vi "TrackExtractor2.vi"() -> ()   [LabVIEW 2012]
panel:
  out "error out":errorcluster
  in  "Tracking file":path=path "C:/Users/Ludovico/Lavoro/Experiments/Autofocus/vermi/track3.txt"
  in  "Positions file":path=path "C:/Users/Ludovico/Lavoro/Experiments/Autofocus/vermi/CONFSTAGELOG/2016_12_16_10_06.txt"
  in  "error in (no error)":errorcluster
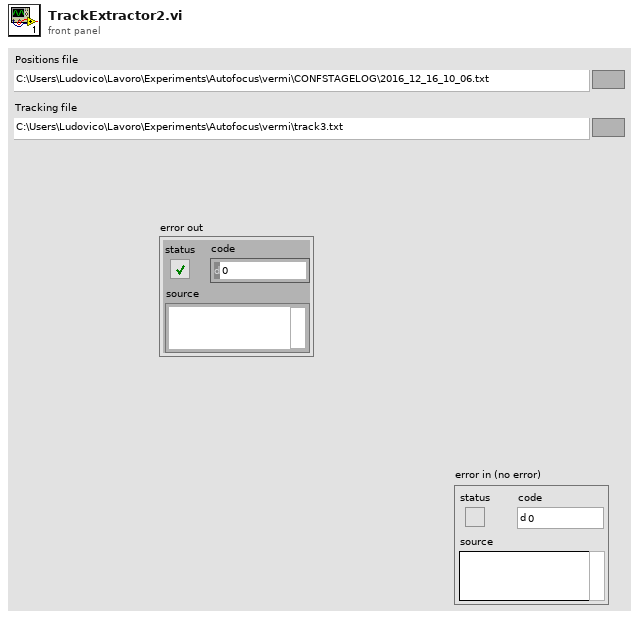
[diagram p1: front panel]
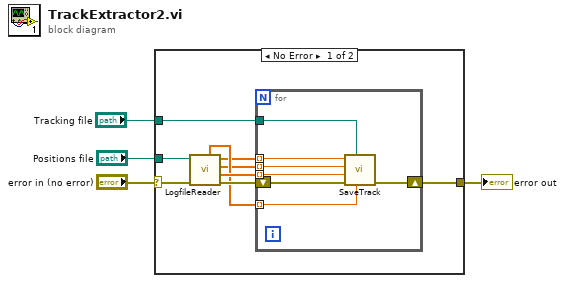
[diagram p0: block diagram]
diagram:
  n1 = case shown="No Error" "error in (no error)" {
    selector: "error in (no error)" -> [w13 w21]
    tunnel: "Positions file" -> [w12 _]
    tunnel: "Tracking file" -> [w6 _]
    tunnel: [w5 w21] -> w1
    frame No Error {
      n2 = call "LogfileReader.vi"("error in (no error)"=w13, "Positions file"=w12) -> ("error out"=w11:errorcluster, "Focus"=w10:dbl[], "Y"=w8:dbl[], "X"=w7:dbl[], "Time"=w9:dbl[])  [unwired: 5 in]
      n3 = for {
        shift-right: [w14] -> w5
        shift-left: w11 -> [w19]
        tunnel: w10 -> [w20] mode=indexing
        tunnel: w9 -> [w18] mode=indexing
        tunnel: w8 -> [w17] mode=indexing
        tunnel: w7 -> [w16] mode=indexing
        tunnel: w6 -> [w15]
        n4 = call "SaveTrack.vi"("Time"=w18, "Track file"=w15, "error in (no error)"=w19, "Focus"=w20, "Y"=w17, "X"=w16) -> ("error out"=w14:errorcluster)  [unwired: 5 in]
      }
    }
    frame Error {
    }
  }
  "error out" <- w1
